vi "Toggle Selection.vi"(8 "error in (no error)":errorcluster, 11 "Shape":refnum<data-value>) -> (0 "error out":errorcluster, 2 "New State":bool, 3 "Shape":refnum<data-value>)   [LabVIEW 2017, in "LV Image Editor Framework.lvlib" / "Selection.lvclass"]
uses:
  Selection.lvclass
  Shape/Shape.lvclass
  Selection.lvclass/Selection.ctl
  Shape/Shape.lvclass/Shape.ctl
  Shape/Read Selectable.vi
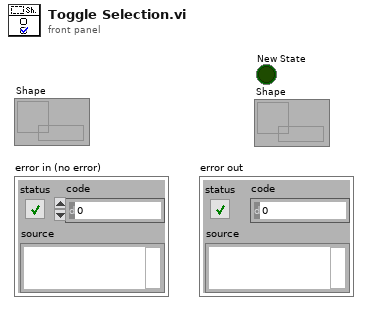
[diagram p1: front panel]
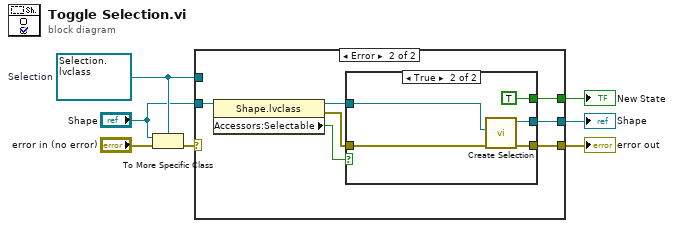
[diagram p0: block diagram]
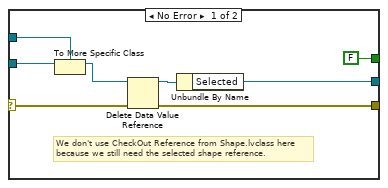
[diagram p2: hidden frame]
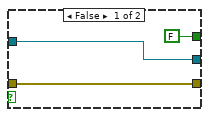
[diagram p3: hidden frame]
diagram:
  w6 = refnum<data-value> refnum  # Selection
  n1 = To More Specific Class(target class=w6, reference="Shape", error in="error in (no error)") -> (error out=w3:errorcluster)  [unwired: 1 out]
  n2 = case shown="Error" w3 {
    selector: w3 -> [w9 _]
    tunnel: [w10 w22] -> w4
    tunnel: [w8 w21] -> w7
    tunnel: w6 -> [w15 _]
    tunnel: "Shape" -> [w14 w20]
    tunnel: [FALSE w17] -> w1
    frame No Error {
      # "We don't use CheckOut Reference from Shape.lvclass here because we still need the selected shape reference."
      n3 = To More Specific Class(target class=w15, reference=w14) -> (specific class reference=w12:refnum<data-value>)  [unwired: 1 in, 1 out]
      n4 = Delete Data Value Reference(data value reference=w12, error in=w9) -> (data value=w11:refnum<class "Selection.lvclass">, error out=w8:errorcluster)
      n5 = Unbundle By Name(w11) -> ("Selected"=w10:refnum<data-value>)
    }
    frame Error {
      n6 = property class="Shape.lvclass"(reference=w20) -> (reference out=w18:refnum<data-value>, error out=w16:errorcluster, "Accessors:Selectable"=w19:bool)  [unwired: 1 in]
      n7 = case shown="True" w19 {
        tunnel: [w25 w30] -> w22
        tunnel: [w23 w29] -> w21
        tunnel: w18 -> [w25 w28]
        tunnel: [FALSE TRUE] -> w17
        tunnel: w16 -> [w23 w26]
        frame False {
        }
        frame True {
          n8 = call "Create Selection.vi"("error in (no error)"=w26, "Shape"=w28) -> ("error out"=w29:errorcluster, "SelectedShape Reference"=w30:refnum<data-value>)  [unwired: 8 in]
        }
      }
    }
  }
  "error out" <- w7
  "New State" <- w1
  "Shape" <- w4
